vi "New Four.vi"() -> ()   [LabVIEW 2015]
doc: "This example VI shows how to convert string data elements to numeric elements so it can be graphed and displayed on an XY Graph."
uses:
  <instrlib>/Keithley 27XX/Public/Configure/Measurement Specific/Configure Thermocouple.vi
  <vilib>/addons/control/pid/pid.llb/PID (DBL).vi
  <instrlib>/Ke24xx/Ke24xx.llb/Ke24xx Configure Source Volt/Cur Level.vi
  <instrlib>/Ke24xx/Ke24xx.llb/Ke24xx Enable/Disable Source Output.vi
  <instrlib>/Keithley 27XX/Keithley 27XX.lvlib
  <vilib>/addons/control/pid/NI_PID_pid.lvlib
  <instrlib>/keithley_24xx/Keithley 24XX/Keithley 24XX.lvlib
panel:
  out "Temp Ch 2 (102 Top)":dbl(graph)
  out "Current out (A)":dbl format="%.2f"
  out "Delta loop 1 (SP - PV)":dbl
  in  "setpoint loop 2":dbl=30.0 format="%.2f"
  in  "PID gains 2400":cluster{"P":dbl, "I":dbl, "D":dbl}={"P"=0.006, "I"=0.02, "D"=0.0} {"D" format="%.3f"; "I" format="%.3f"; "P" format="%.3f"}
  in  "Current range":cluster{"output high":dbl, "output low":dbl}={"output high"=1.0, "output low"=-1.0} {"output low" format="%.2f"; "output high" format="%.2f"}
  out "error out 2400":errorcluster
  in  "Loop 1":bool=TRUE
  in  "Voltage":dbl=2.1
  in  "Source Mode  (0: Voltage)":u16(ring)=1 items=["Voltage", "Current"]
  in  "Displayed Measurement (0: Voltage)":u16(ring)=1 items=["Voltage", "Current", "Resistance"]
  in  "Voltage Limit (12 V)":dbl=12.0 format="%.2g"
  in  "Output":u16(ring) items=["Volts", "Current", "Resistance"]
  in  "Enable Auto Range (T:Enable)":bool=TRUE
  in  "Manual Range (1.0)":dbl
  in  "VISA resource name":refnum<visa-resource-name>="GPIB0::2::INSTR"
  out "Temp Ch 4 (104 PID 2)":dbl(graph)
  out "Delta loop 2":dbl
  in  "setpoint loop 1":dbl=30.0 format="%.2f"
  in  "Voltage range":cluster{"output high":dbl, "output low":dbl}={"output high"=12.0, "output low"=-12.0} {"output low" format="%.2f"; "output high" format="%.2f"}
  in  "PID gains 2425":cluster{"P":dbl, "I":dbl, "D":dbl}={"P"=0.01, "I"=0.007, "D"=0.0} {"D" format="%.3f"; "I" format="%.3f"; "P" format="%.3f"}
  out "Voltage out (V)":dbl
  in  "Current":dbl=1.0 min=-1100.0 max=1100.0 step=1.0 format="%.2p"
  in  "Loop 2":bool
  in  "?":path=path "C:/Users/Guest_2/Desktop/Zong Long/Data trial.txt"
  in  "Save File?":bool
  in  "format string":string
  in  "delimiter (Tab)":string
  out "Data":string
  out "Voltage 2":dbl(graph)
  out "Voltage 1":dbl(graph)
  out "Temperature Ch 1 (101 Bot)":dbl(graph)
  out "Temperature Ch 3 (103 PID 1)":dbl(graph)
  out "Iteration":i32
  out "Time elapsed":dbl
  in  "Pause/Continue":bool
  out "error out 2425":errorcluster
  in  "range":i32
  in  "function":i32(slide)
  in  "error in (no error) 2":errorcluster
  in  "reset device":u16(slide)=1
  in  "id query":u16(slide)=1
  in  "resource name":string="GPIB0::20::INSTR"
  out "Temp Ch 4":dbl
  out "Temp Ch 2":dbl
  out "Temp Ch 3":dbl
  out "Temperature Ch 1 (101 Top)":dbl
  out "Voltage Ch 1":dbl
  out "Voltage Ch 2":dbl
  in  "stop":bool
  in  "Number of channels 2":i32=2
  in  "Function (0: DC Voltage)":u16(ring) items=["DC Voltage", "AC Voltage", "DC Current", "AC Current", "Resistance", "Four-Wire Resistance", "Temperature (C)", "Frequency", "Period", "Continuity"]
  in  "Channel List (101) 2":string="101:102"
  in  "Serial Configuration 2":T1={"Baud Rate (9600)"=9600, "Flow Control (1: XON/XOFF)"=1, "Termination Char (0:CR)"=0} {"Termination Char (0:CR)" items=["CR", "LF", "CRLF (Do not use)", "LFCR (Do not use)"]; "Flow Control (1: XON/XOFF)" items=["None", "XON/XOFF", "RTS/CTS (2701 Only)", "XON/XOFF & RTS/CTS (2701 Only)"]; "Baud Rate (9600)" items=["300"=300, "600"=600, "1200"=1200, "2400"=2400, "4800"=4800, "9600"=9600, "19.2k"=19200, "38.4k (2701 Only)"=38400, "57.6k (2701 Only)"=57600, "115.2k (2701 Only)"=115200]}
  in  "Keithley VISA resource name 2":refnum<visa-resource-name>="GPIB0::16::INSTR"
  in  "Enable Open Detector? (False)":bool=TRUE
  in  "Simulated Reference Temperature (23 deg C)":dbl=23.0
  in  "Reference Junction Type (1: Internal)":u16(ring)=1 items=["Simulated", "Internal", "External"]
  in  "Thermocouple Type (1: K)":u16(ring)=1 items=["J", "K", "T", "E", "R", "S", "B", "N"]
  in  "Number of channels":i32=4
  in  "Function (6: Temp)":u16(ring)=6 items=["DC Voltage", "AC Voltage", "DC Current", "AC Current", "Resistance", "Four-Wire Resistance", "Temperature (C)", "Frequency", "Period", "Continuity"]
  in  "Channel List (101)":string="101:104"
  in  "Serial Configuration":T1={"Baud Rate (9600)"=9600, "Flow Control (1: XON/XOFF)"=1, "Termination Char (0:CR)"=0} {"Termination Char (0:CR)" items=["CR", "LF", "CRLF (Do not use)", "LFCR (Do not use)"]; "Flow Control (1: XON/XOFF)" items=["None", "XON/XOFF", "RTS/CTS (2701 Only)", "XON/XOFF & RTS/CTS (2701 Only)"]; "Baud Rate (9600)" items=["300"=300, "600"=600, "1200"=1200, "2400"=2400, "4800"=4800, "9600"=9600, "19.2k"=19200, "38.4k (2701 Only)"=38400, "57.6k (2701 Only)"=57600, "115.2k (2701 Only)"=115200]}
  in  "Keithley VISA resource name":refnum<visa-resource-name>="GPIB0::19::INSTR"
  # "Keithley 2425 INIT,\nLoop 1 ch(2,3)"
  # "Keithley 2400 INIT,\nLoop 2 (ch1, 4)"
  # "File INIT"
  # "2700 Temp INIT"
  # "2700 Voltage INIT"
  # "Operations"
  # "Note: Always remember\nto turn off Loop  output before STOP"
  # "Data"
  # "Loop 1 (Top)"
  # "Loop 2 (Bot)"
  # "General"
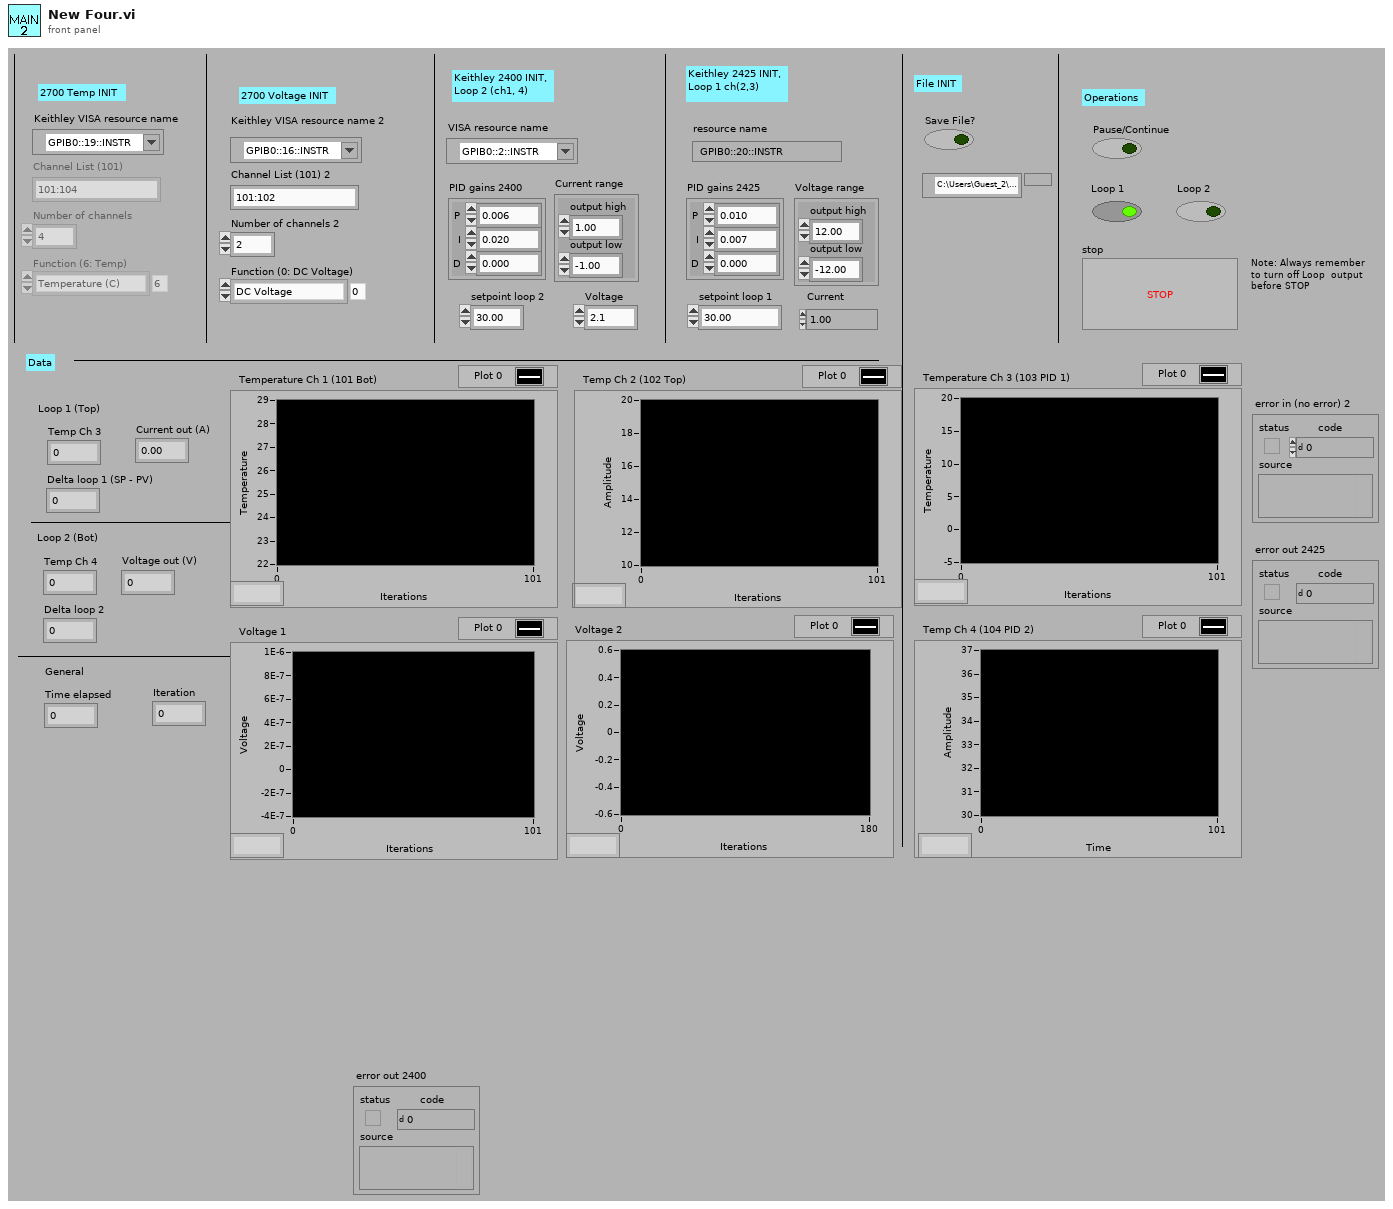
[diagram p1: front panel]
types:
  T1 = cluster{"Baud Rate (9600)":u32, "Flow Control (1: XON/XOFF)":u16, "Termination Char (0:CR)":u16}
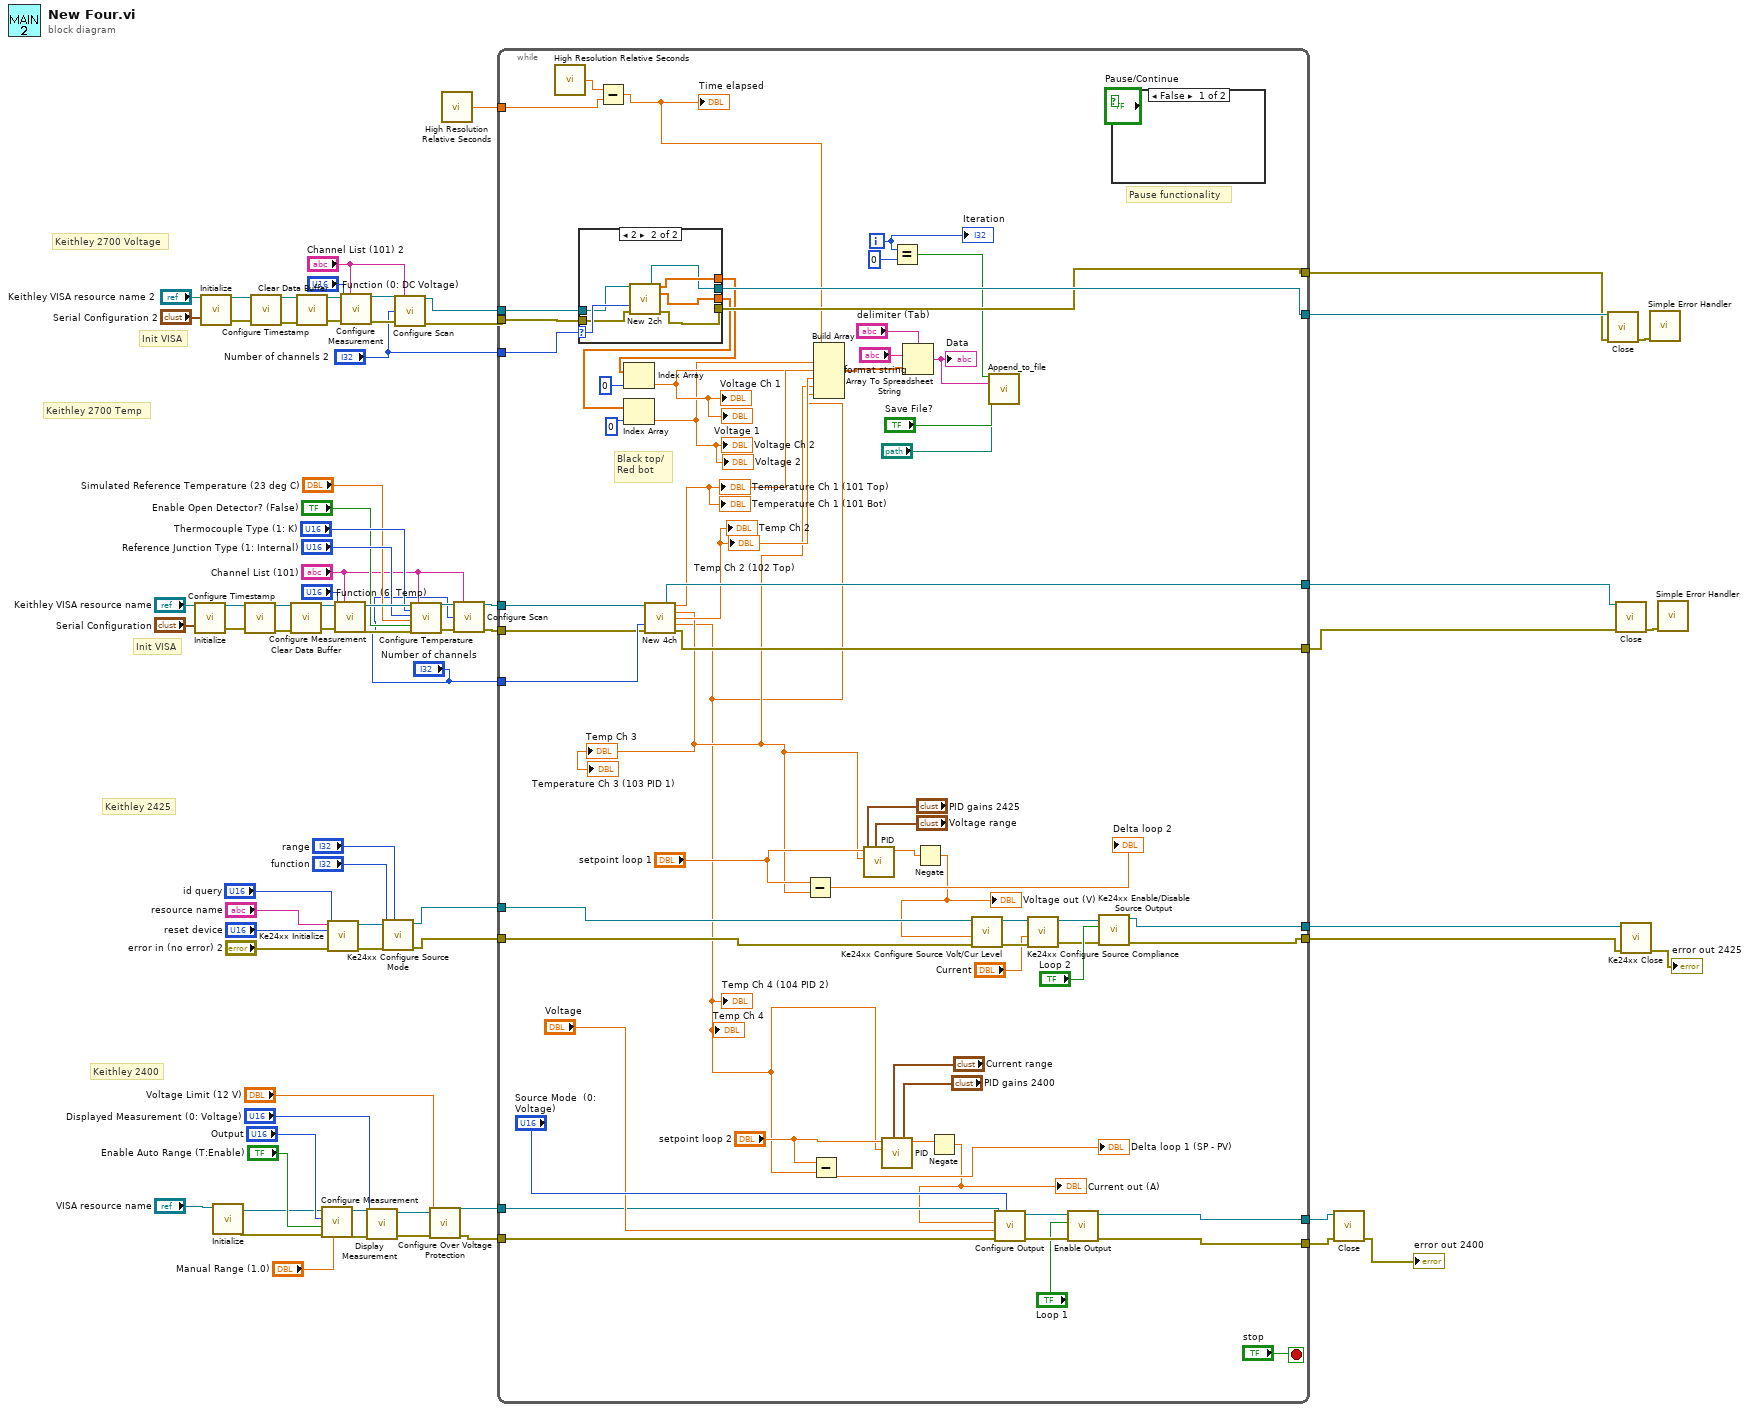
[diagram p0: block diagram]
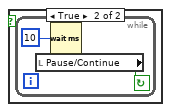
[diagram p2: hidden frame]
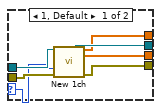
[diagram p3: hidden frame]
diagram:
  # "Keithley 2400"
  # "Keithley 2425"
  # "Keithley 2700 Voltage"
  # "Init VISA"
  # "Keithley 2700 Temp"
  # "Init VISA"
  n1 = call <instrlib>:"Initialize.vi"("VISA resource name"="Keithley VISA resource name", "Serial Configuration"="Serial Configuration") -> ("VISA resource name out"=w71:refnum<visa-resource-name>, "error out"=w70:errorcluster)  [unwired: 12 in]
  n2 = call <instrlib>:"Initialize.vi"("VISA resource name"="Keithley VISA resource name 2", "Serial Configuration"="Serial Configuration 2") -> ("VISA resource name out"=w53:refnum<visa-resource-name>, "error out"=w52:errorcluster)  [unwired: 12 in]
  n3 = call <instrlib>:"Initialize.vi"("VISA resource name"="VISA resource name") -> ("error out"=w12:errorcluster, "VISA resource name out"=w13:refnum<visa-resource-name>)  [unwired: 9 in]
  n4 = call <instrlib>:"Configure Timestamp.vi"("VISA resource name"=w71, "error in (no error)"=w70) -> ("VISA resource name out"=w68:refnum<visa-resource-name>, "error out"=w67:errorcluster)  [unwired: 12 in]
  n5 = call <instrlib>:"Configure Timestamp.vi"("VISA resource name"=w53, "error in (no error)"=w52) -> ("VISA resource name out"=w50:refnum<visa-resource-name>, "error out"=w49:errorcluster)  [unwired: 12 in]
  n6 = call <instrlib>:"Clear Data Buffer.vi"("VISA resource name"=w68, "error in (no error)"=w67) -> ("VISA resource name out"=w66:refnum<visa-resource-name>, "error out"=w69:errorcluster)  [unwired: 12 in]
  n7 = call <instrlib>:"Clear Data Buffer.vi"("VISA resource name"=w50, "error in (no error)"=w49) -> ("VISA resource name out"=w48:refnum<visa-resource-name>, "error out"=w51:errorcluster)  [unwired: 12 in]
  n8 = call <instrlib>:"Configure Measurement.vi"("Manual Range (1.0)"="Manual Range (1.0)", "error in (no error)"=w12, "Enable Auto Range (T:Enable)"="Enable Auto Range (T:Enable)", "Function (0: Volts)"="Output", "VISA resource name"=w13) -> ("error out"=w10:errorcluster, "VISA resource name out"=w11:refnum<visa-resource-name>)  [unwired: 5 in]
  n9 = call <instrlib>:"Ke24xx Initialize.vi"("error in (no error)"="error in (no error) 2", "reset device"="reset device", "id query"="id query", "resource name"="resource name") -> ("error out"=w26:errorcluster, "instrument handle out"=w27:refnum<visa-resource-name>)  [unwired: 5 in, 1 out]
  n10 = call <instrlib>:"Configure Measurement.vi"("VISA resource name"=w66, "Scan List (Empty)"="Channel List (101)", "Function (0: DC Voltage)"="Function (6: Temp)", "error in (no error)"=w69) -> ("VISA resource name out"=w64:refnum<visa-resource-name>, "error out"=w61:errorcluster)  [unwired: 10 in]
  n11 = call <instrlib>:"Configure Measurement.vi"("VISA resource name"=w48, "Scan List (Empty)"="Channel List (101) 2", "Function (0: DC Voltage)"="Function (0: DC Voltage)", "error in (no error)"=w51) -> ("VISA resource name out"=w46:refnum<visa-resource-name>, "error out"=w45:errorcluster)  [unwired: 10 in]
  n12 = call <instrlib>:"Display Measurement.vi"("error in (no error)"=w10, "Displayed Measurement (0: Voltage)"="Displayed Measurement (0: Voltage)", "VISA resource name"=w11) -> ("error out"=w8:errorcluster, "VISA resource name out"=w9:refnum<visa-resource-name>)  [unwired: 7 in]
  n13 = call <instrlib>:"Ke24xx Configure Source Mode.vi"("range"="range", "error in (no error)"=w26, "function"="function", "instrument handle"=w27) -> ("error out"=w21:errorcluster, "instrument handle out"=w20:refnum<visa-resource-name>)  [unwired: 5 in, 1 out]
  n14 = call <instrlib>:"Configure Scan.vi"("VISA resource name"=w46, "Channel List (101:110)"="Channel List (101) 2", "Sample Count (100)"="Number of channels 2", "error in (no error)"=w45) -> ("VISA resource name out"=w43:refnum<visa-resource-name>, "error out"=w42:errorcluster)  [unwired: 10 in]
  n15 = call-poly <instrlib>:"Configure Temperature.vi"("VISA resource name"=w64, "Thermocouple Type (1: K)"="Thermocouple Type (1: K)", "Reference Junction Type (0: Simulated)"="Reference Junction Type (1: Internal)", "Simulated Reference Temperature (23 deg C)"="Simulated Reference Temperature (23 deg C)", "Enable Open Detector? (False)"="Enable Open Detector? (False)", "error in (no error)"=w61, "Scan List (Empty)"="Channel List (101)") -> ("VISA resource name out"=w63:refnum<visa-resource-name>, "error out"=w62:errorcluster)  [unwired: 11 in]
  n16 = call <instrlib>:"Configure Over Voltage Protection.vi"("error in (no error)"=w8, "Voltage Limit (0.0 V)"="Voltage Limit (12 V)", "VISA resource name"=w9) -> ("error out"=w4:errorcluster, "VISA resource name out"=w5:refnum<visa-resource-name>)  [unwired: 7 in]
  n17 = call <vilib>:"High Resolution Relative Seconds.vi"() -> ("relative seconds"=w18:dbl)
  n18 = call <instrlib>:"Configure Scan.vi"("VISA resource name"=w63, "Channel List (101:110)"="Channel List (101)", "Sample Count (100)"="Number of channels", "error in (no error)"=w62) -> ("VISA resource name out"=w41:refnum<visa-resource-name>, "error out"=w40:errorcluster)  [unwired: 10 in]
  n19 = while {
    tunnel: w43 -> [w137]
    tunnel: w42 -> [w136]
    tunnel: w41 -> [w128]
    tunnel: w40 -> [w126]
    tunnel: "Number of channels" -> [w127]
    tunnel: "Number of channels 2" -> [w135]
    tunnel: [w134] -> w35
    tunnel: [w133] -> w34
    tunnel: [w124] -> w33
    tunnel: [w125] -> w32
    tunnel: [w99] -> w22
    tunnel: w21 -> [w98]
    tunnel: w20 -> [w101]
    tunnel: [w100] -> w19
    tunnel: w18 -> [w121]
    tunnel: w5 -> [w88]
    tunnel: w4 -> [w87]
    tunnel: [w86] -> w2
    tunnel: [w85] -> w1
    i -> [w110]
    stop <- "stop" stop-if-true
    # "Black top/\nRed bot"
    # "Pause functionality"
    n20 = call <vilib>:"High Resolution Relative Seconds.vi"() -> ("relative seconds"=w122:dbl)
    n21 = case shown="2" w135 {
      selector: w135 -> [w145 w154]
      tunnel: w137 -> [w147 w152]
      tunnel: w136 -> [w146 w153]
      tunnel: [w144 w148] -> w134
      tunnel: [w143 w150] -> w133
      tunnel: [w142 w151] -> w129
      tunnel: [w141 w149] -> w131
      frame 1, Default {
        n22 = call "New 1ch.vi"("VISA resource name out"=w147, "Number of channels"=w145, "error out"=w146) -> ("VISA resource name out 2"=w144:refnum<visa-resource-name>, "Array 2"=w142:dbl[], "Array"=w141:dbl[], "error out 2"=w143:errorcluster)  [unwired: 9 in]
      }
      frame 2 {
        n23 = call "New 2ch.vi"("VISA resource name out"=w152, "Number of channels"=w154, "error out"=w153) -> ("VISA resource name out 2"=w148:refnum<visa-resource-name>, "Array 2"=w151:dbl[], "Array"=w149:dbl[], "error out 2"=w150:errorcluster)  [unwired: 9 in]
      }
    }
    n24 = Subtract(x=w122, y=w121) -> (x-y=w120:dbl)
    "Time elapsed" <- w120
    n25 = Index Array(array=w129, index=0) -> (element=w118:dbl)
    "Voltage Ch 1" <- w118
    "Voltage 1" <- w118
    n26 = Index Array(array=w131, index=0) -> (element=w117:dbl)
    "Voltage Ch 2" <- w117
    "Voltage 2" <- w117
    n27 = call "New 4ch.vi"("VISA resource name out"=w128, "Number of channels"=w127, "error out"=w126) -> ("VISA resource name out 2"=w125:refnum<visa-resource-name>, "element"=w119:dbl, "element 2"=w75:dbl, "element 3"=w80:dbl, "element 4"=w74:dbl, "error out 2"=w124:errorcluster)  [unwired: 7 in]
    "Temperature Ch 1 (101 Top)" <- w119
    "Temp Ch 3" <- w75
    "Temp Ch 2" <- w80
    "Temp Ch 4" <- w74
    "Temperature Ch 3 (103 PID 1)" <- w75
    "Temperature Ch 1 (101 Bot)" <- w119
    "Temp Ch 4 (104 PID 2)" <- w74
    "Temp Ch 2 (102 Top)" <- w80
    n28 = Subtract(x="setpoint loop 1", y=w75) -> (x-y=→"Delta loop 2":dbl)
    n29 = Subtract(x="setpoint loop 2", y=w74) -> (x-y=→"Delta loop 1 (SP - PV)":dbl)
    n30 = Build Array(w120, w118, w117, w119, w80, w75, w74) -> (w116:dbl[])
    n31 = call-poly <vilib>:"PID.vi"("output range"="Voltage range", "PID gains"="PID gains 2425", "process variable"=w75, "setpoint"="setpoint loop 1") -> ("output"=w77:dbl)  [unwired: 6 in, 1 out]
    n32 = call-poly <vilib>:"PID.vi"("output range"="Current range", "PID gains"="PID gains 2400", "process variable"=w74, "setpoint"="setpoint loop 2") -> ("output"=w79:dbl)  [unwired: 6 in, 1 out]
    n33 = Equal?(x=w110, y=0) -> (x = y?=w108:bool)
    n34 = Array To Spreadsheet String(delimiter (Tab)="delimiter (Tab)", array=w116, 3:"format string") -> (spreadsheet string=w113:string)
    "Data" <- w113
    n35 = Negate(x=w77) -> (-x=w76:dbl)
    "Voltage out (V)" <- w76
    n36 = Negate(x=w79) -> (-x=w78:dbl)
    "Current out (A)" <- w78
    n37 = call "Ke24xx Configure Source Volt/Cur Level.vi"("error in (no error)"=w98, "level"=w76, "instrument handle"=w101) -> ("error out"=w105:errorcluster, "instrument handle out"=w106:refnum<visa-resource-name>)  [unwired: 6 in, 1 out]
    n38 = call "Append_to_file.vi"("Boolean"=w108, "text"=w113, "Save File?"="Save File?", "file path (use dialog)"="?") -> ()  [unwired: 11 in, 1 out]
    n39 = call <instrlib>:"Configure Output.vi"("Source Mode  (0: Voltage)"="Source Mode  (0: Voltage)", "error in (no error)"=w87, "Compliance  Level (0.1)"="Voltage", "Output Level (0)"=w78, "VISA resource name"=w88) -> ("error out"=w90:errorcluster, "VISA resource name out"=w91:refnum<visa-resource-name>)  [unwired: 5 in]
    n40 = call <instrlib>:"Ke24xx Configure Source Compliance.vi"("error in (no error)"=w105, "level"="Current", "instrument handle"=w106) -> ("error out"=w103:errorcluster, "instrument handle out"=w104:refnum<visa-resource-name>)  [unwired: 6 in, 1 out]
    n41 = call <instrlib>:"Enable Output.vi"("error in (no error)"=w90, "Enable Output (T: Enable)"="Loop 1", "VISA resource name"=w91) -> ("error out"=w85:errorcluster, "VISA resource name out"=w86:refnum<visa-resource-name>)  [unwired: 7 in]
    n42 = call "Ke24xx Enable/Disable Source Output.vi"("error in (no error)"=w103, "state"="Loop 2", "instrument handle"=w104) -> ("error out"=w99:errorcluster, "instrument handle out"=w100:refnum<visa-resource-name>)  [unwired: 6 in, 1 out]
    n43 = case shown="False" "Pause/Continue" {
      frame False {
      }
      frame True {
        n44 = while {
          stop <- w140 continue-if-true
          n45 = local read "Pause/Continue"() -> (w140:bool)
          n46 = Wait (ms)(milliseconds to wait=u32 10) -> ()  [unwired: 1 out]
        }
      }
    }
    "Iteration" <- w110
  }
  n47 = call <instrlib>:"Close.vi"("error in (no error)"=w1, "VISA resource name"=w2) -> ("error out"=→"error out 2400":errorcluster)  [unwired: 9 in]
  n48 = call <instrlib>:"Close.vi"("VISA resource name"=w35, "error in (no error)"=w34) -> ("error out"=w37:errorcluster)  [unwired: 13 in]
  n49 = call <instrlib>:"Close.vi"("VISA resource name"=w32, "error in (no error)"=w33) -> ("error out"=w36:errorcluster)  [unwired: 13 in]
  n50 = call <instrlib>:"Ke24xx Close.vi"("error in (no error)"=w22, "instrument handle"=w19) -> ("error out"=→"error out 2425":errorcluster)  [unwired: 8 in, 1 out]
  n51 = call <vilib>:"Simple Error Handler.vi"("error in (no error)"=w37) -> ()  [unwired: 4 in, 5 out]
  n52 = call <vilib>:"Simple Error Handler.vi"("error in (no error)"=w36) -> ()  [unwired: 4 in, 5 out]
